vi "UserinterfaceExpert.vi"() -> ()   [LabVIEW 2023]
panel:
  in  "Level":dbl(slide) scale=0.0..120.0
  in  "?":bool
  out "LED 1 (25 %)":bool
  out "LED 2 (50 %)":bool
  out "LED 3 (75%)":bool
  out "LED 4 (100%)":bool
  out "?":dbl
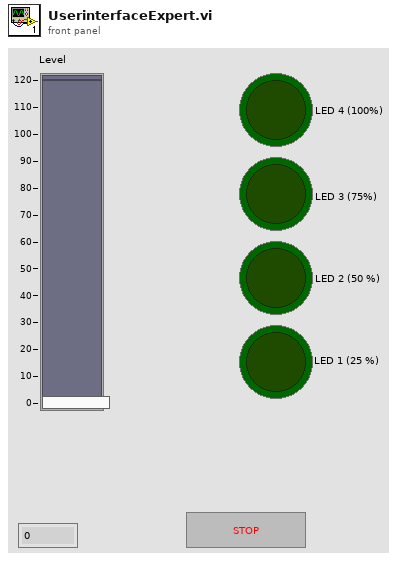
[diagram p1: front panel]
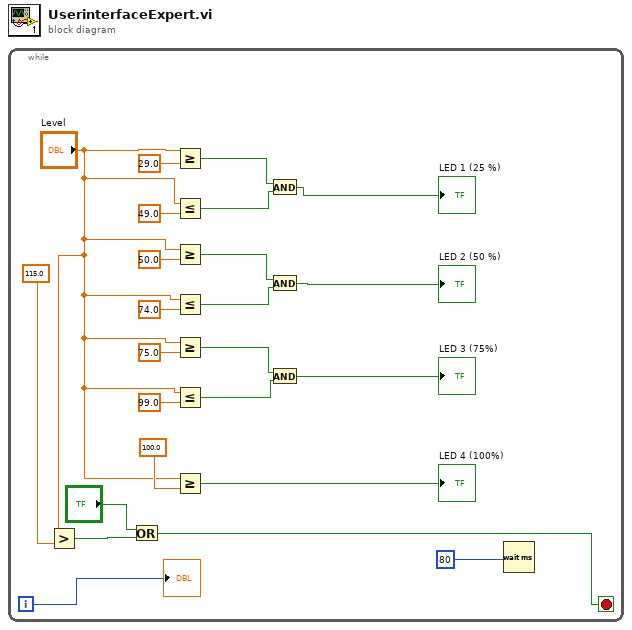
[diagram p0: block diagram]
diagram:
  n1 = while {
    i -> [w20]
    stop <- w21 stop-if-true
    n2 = Greater?(x="Level", y=115.0) -> (0:w22:bool)
    n3 = Or(x="?", y=w22) -> (x .or. y?=w21:bool)
    n4 = Greater Or Equal?(x="Level", y=29.0) -> (x >= y?=w17:bool)
    n5 = Less Or Equal?(x="Level", y=49.0) -> (x <= y?=w16:bool)
    n6 = Greater Or Equal?(x="Level", y=50.0) -> (x >= y?=w12:bool)
    n7 = Less Or Equal?(x="Level", y=74.0) -> (x <= y?=w11:bool)
    n8 = Greater Or Equal?(x="Level", y=75.0) -> (x >= y?=w7:bool)
    n9 = Less Or Equal?(x="Level", y=99.0) -> (x <= y?=w6:bool)
    n10 = Greater Or Equal?(x="Level", y=100.0) -> (x >= y?=→"LED 4 (100%)":bool)
    n11 = And(x=w17, y=w16) -> (x .and. y?=→"LED 1 (25 %)":bool)
    n12 = And(x=w12, y=w11) -> (x .and. y?=→"LED 2 (50 %)":bool)
    n13 = And(x=w7, y=w6) -> (x .and. y?=→"LED 3 (75%)":bool)
    n14 = Wait (ms)(milliseconds to wait=u32 80 ("millisecond timer value")) -> ()  [unwired: 1 out]
    "?" <- w20
  }
